vi "Main_FFT.vi"() -> ()   [LabVIEW 2026]
doc: "This template is for the Queued Message Handler design pattern.\n\nThe Event Handling Loop generates messages based on user interface actions.\n\nThe Message Handling Loop processes messages generated by the Event Handling Loop, or by other messages. The messages are string values, so new messages can be added easily to the Message Cases case structure in the Message Handling Loop. Each message cluster can also provide an optional value for Message Data, which is a variant that can be converted to whatever message-specific data is required."
uses:
  SubVIs/Controls/PCO_Config.ctl
  SubVIs/Controls/UI Data.ctl
  SubVIs/pco.labview/camera/Camera.lvclass
  SubVIs/Controls/TypeDef_FGV.ctl
  SubVIs/QMH/Message Queue/Enqueue Message (Single).vi
  SubVIs/QMH/Message Queue/Message Queue.lvlib
  SubVIs/QMH/User Event - Stop/User Event - Stop.lvlib
  SubVIs/pco.labview/pco.sdk/TimingControl/TimingControl.lvlib
panel:
  out "FFT":T1(plugin-control)
  out "Camera":T1(plugin-control)
  in  "# of frames":u16=100
  in  "SavePath":path=path "E:/exp_data/Seb"
  in  "Binning for FFT":u16(ring)=8 items=["1x1"=1, "2x2"=2, "4x4"=4, "8x8"=8]
  in  "Stop live":bool
  in  "FFT?":bool=TRUE
  in  "Grab":bool
  in  "Live":bool
  in  "PCO_Config":T2={"Exposure time (s)"=0.01, "TriggerMode"=0, "ROI X0"=1, "ROI Y0"=1, "ROI X1"=2048, "ROI Y1"=2048, "Binning"=1} {"TriggerMode" items=["auto sequence", "software trigger", "external exposure start", "external exposure control"]}
  out "Current task":string="\"Exit\" button pressed"
  in  "Exit":bool
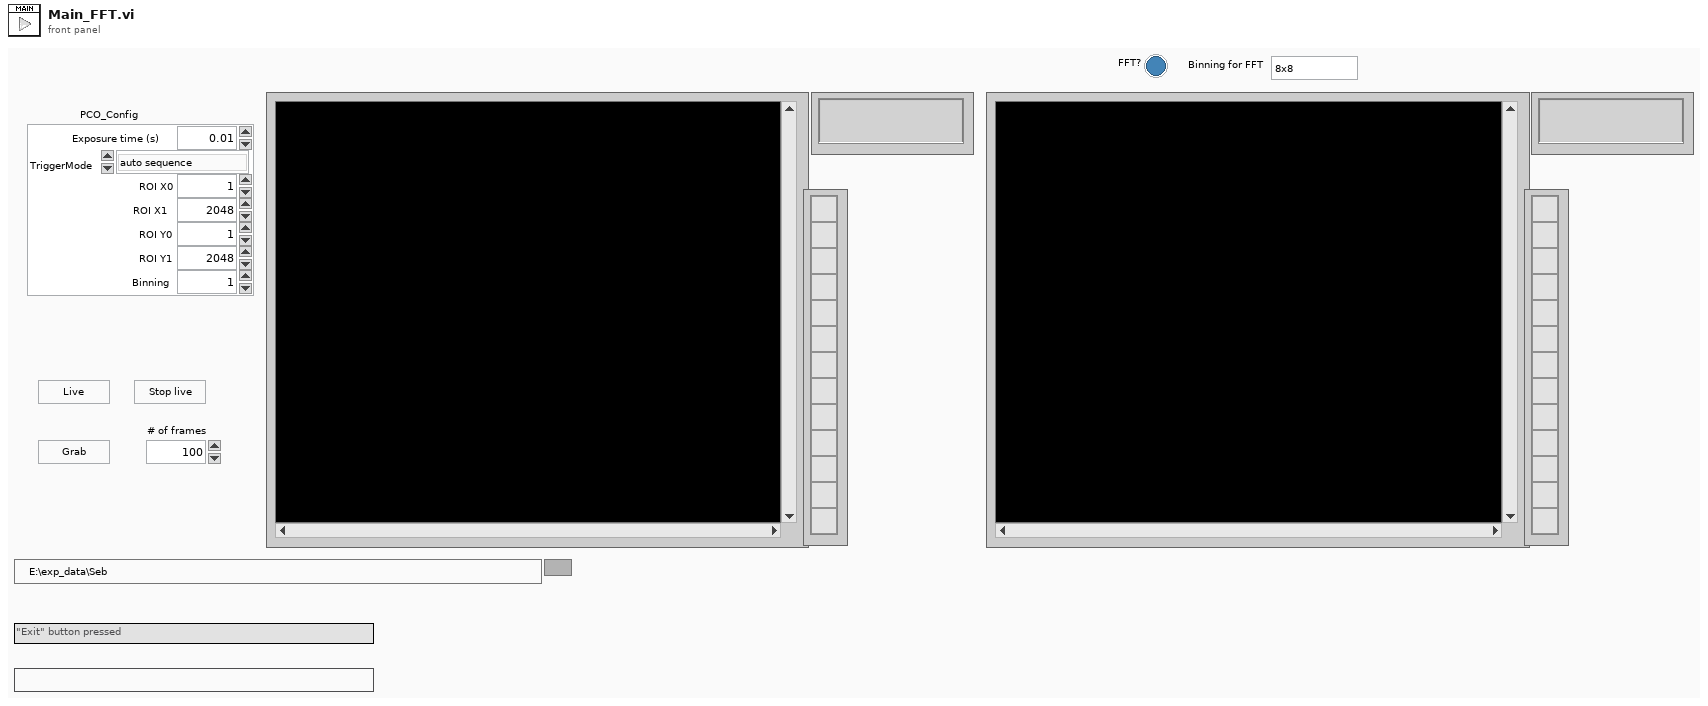
[diagram p1: front panel]
types:
  T1 = typedef "IMAQ Image.ctl" = refnum<image>
  T2 = typedef "PCO_Config.ctl" = cluster{"Exposure time (s)":dbl, "TriggerMode":u16, "ROI X0":u16, "ROI Y0":u16, "ROI X1":u16, "ROI Y1":u16, "Binning":u8}
  T3 = typedef "UI Data.ctl" = cluster{"Data Display Ref":refnum<vi>, "Exit Button Ref":refnum<vi>, "Message":string}
  T4 = typedef "Message Queue.lvlib/All Message Queues.ctl" = cluster{"UI":refnum<queue>, "Camera loop":refnum<queue>, "Display loop":refnum<queue>}
  T5 = typedef "TypeDef_FGV.ctl" = enum16{"Initialize", "Write", "Read"}
  T6 = typedef "Image Type" = u32
  T7 = enum16{"auto sequence", "software trigger", "external exposure start", "external exposure control"}
  T8 = typedef "Camera.lvclass/binning.ctl" = cluster{"vert":u16, "horz":u16, "mode":u16}
  T9 = cluster{"exposure_time_s":dbl, "delay_time_s":dbl, "roi":cluster{"x0":u64, "y0":u64, "x1":u64, "y1":u64}, "timestamp_mode":u16, "pixelrate":u32, "conversion_factor":sgl, "trigger_mode":u16, "acquire_mode":u16, "acquire_sequence_number":u32, "metadata_mode":u16, "noisefilter_mode":u16, "pixel_format":u32, "binning":T8, "auto_exposure":cluster{"region":u16, "min_exposure_s":dbl, "max_exposure_s":dbl}}
  T10 = cluster{"wSignalNum":u16, "wEnabled":u16, "wType":u16, "wPolarity":u16, "wFilterSetting":u16, "wSelected":u16, "dwParameter":u32[], "dwSignalFunctionality":u32[]}
  T11 = cluster{"wVersion":u16, "dwIMAGE_COUNTER":u32, "dwIMAGE_TIME_US":u32, "lvTimestamp":timestamp, "bIMAGE_TIME_STATUS":u8, "wEXPOSURE_TIME_BASE":u16, "dwEXPOSURE_TIME":u32, "dwFRAMERATE_MILLIHZ":u32, "sSENSOR_TEMPERATURE":i16, "wIMAGE_SIZE_X":u16, "wIMAGE_SIZE_Y":u16, "bBINNING_X":u8, "bBINNING_Y":u8, "dwSENSOR_READOUT_FREQUENCY":u32, "wSENSOR_CONV_FACTOR":u16, "dwCAMERA_SERIAL_NO":u32, "wCAMERA_TYPE":u16, "bBIT_RESOLUTION":u8, "bSYNC_STATUS":u8, "wDARK_OFFSET":u16, "bTRIGGER_MODE":u8, "bDOUBLE_IMAGE_MODE":u8, "bCAMERA_SYNC_MODE":u8, "bIMAGE_TYPE":u8, "wCOLOR_PATTERN":u16, "wCAMERA_SUBTYPE":u16, "dwEVENT_NUMBER":u32, "wIMAGE_SIZE_X_Offset":u16, "wIMAGE_SIZE_Y_Offset":u16, "bREADOUT_MODE":u8}[]
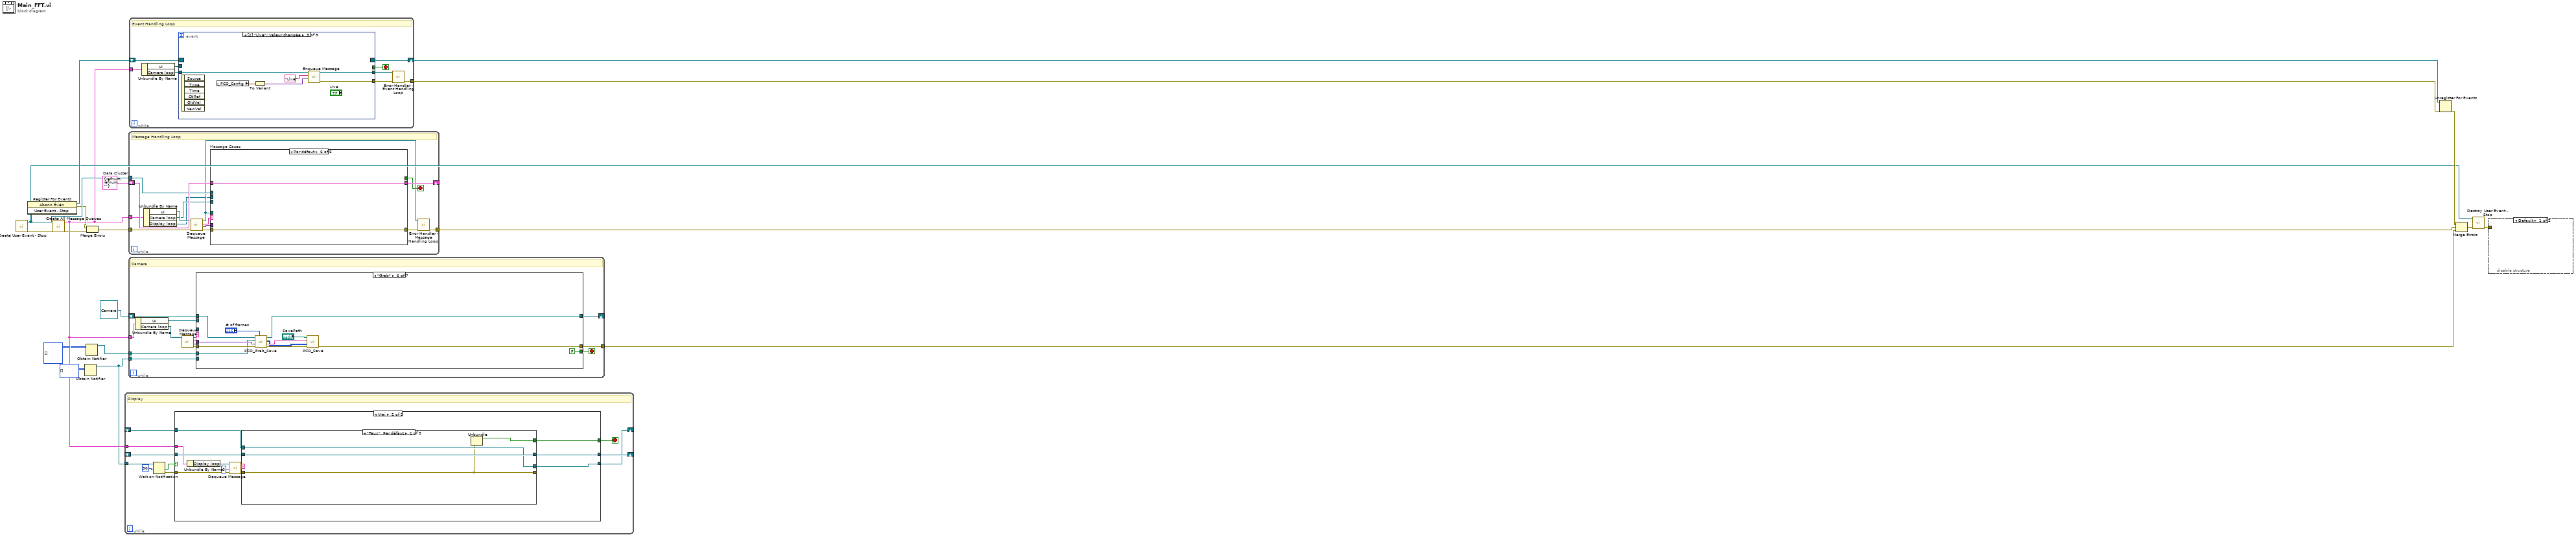
[diagram p0: block diagram]
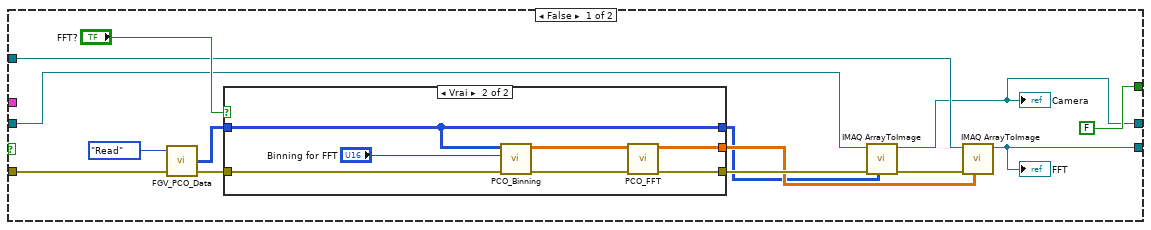
[diagram p2: hidden frame]
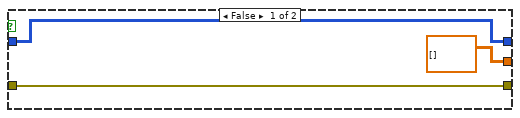
[diagram p3: hidden frame]
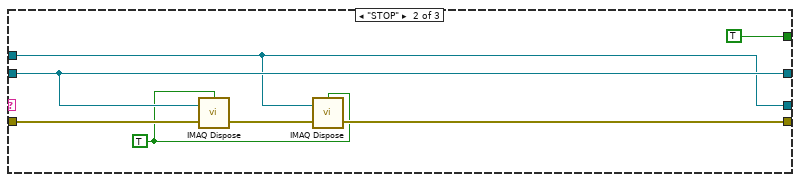
[diagram p4: hidden frame]
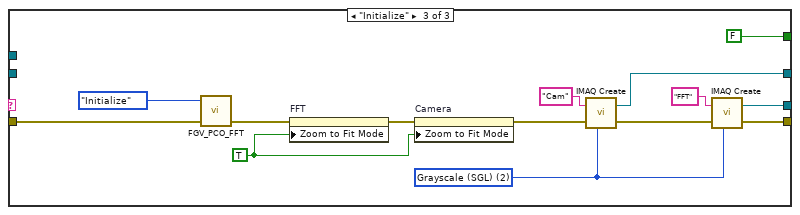
[diagram p5: hidden frame]
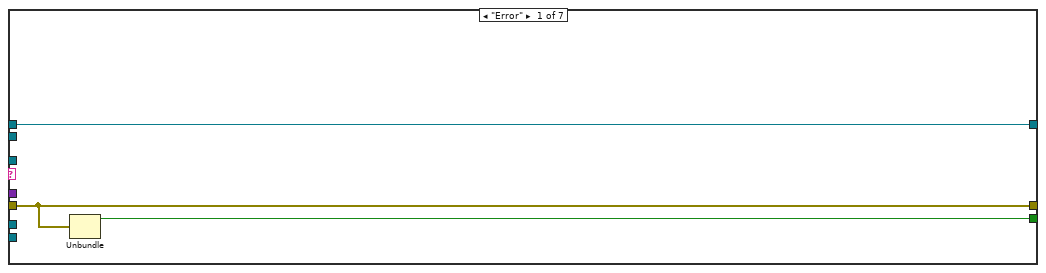
[diagram p6: hidden frame]
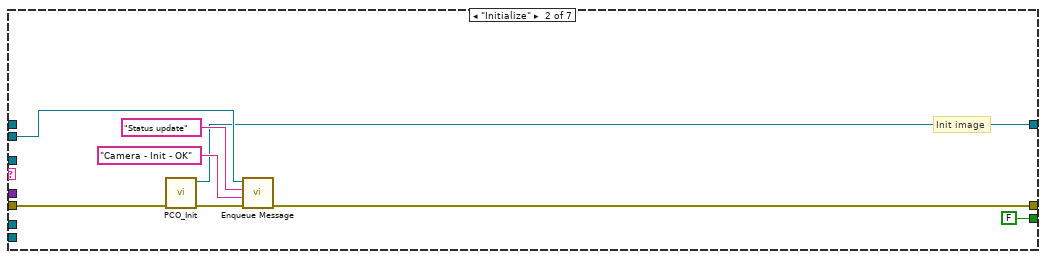
[diagram p7: hidden frame]
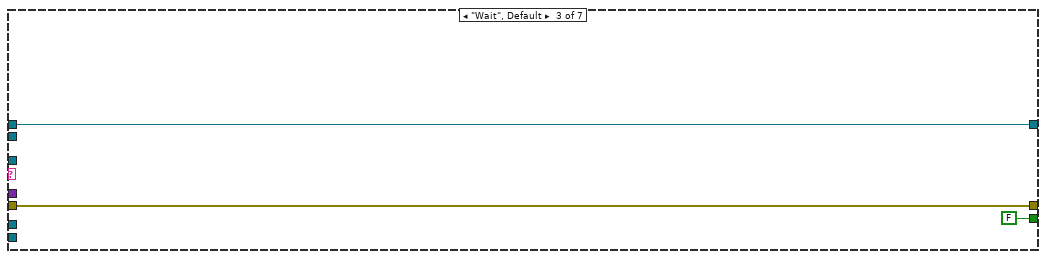
[diagram p8: hidden frame]
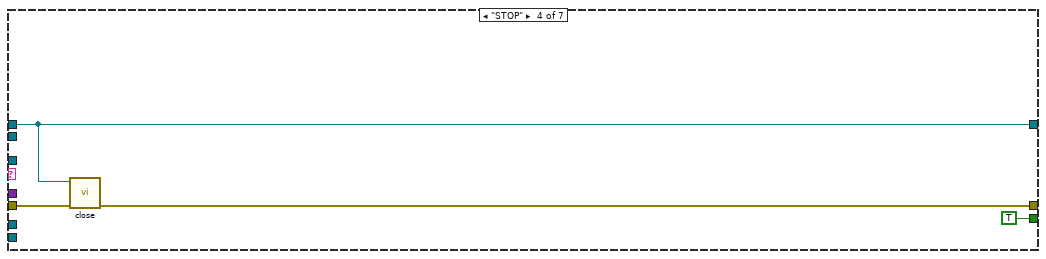
[diagram p9: hidden frame]
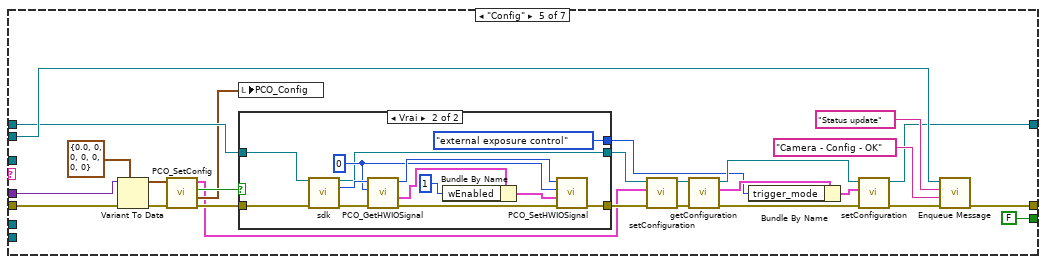
[diagram p10: hidden frame]
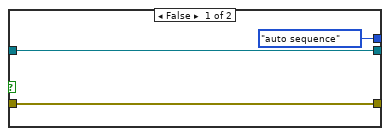
[diagram p11: hidden frame]
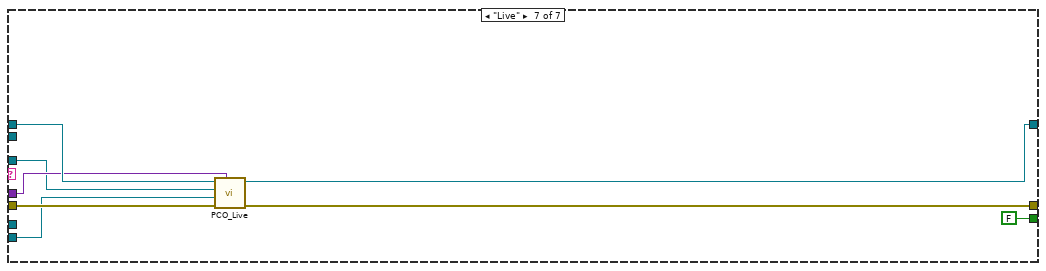
[diagram p12: hidden frame]
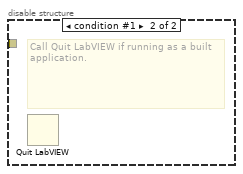
[diagram p13: hidden frame]
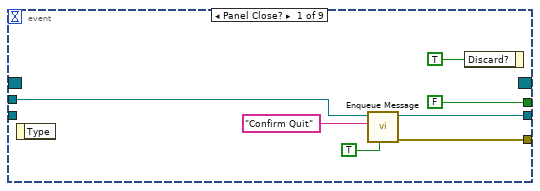
[diagram p14: hidden frame]
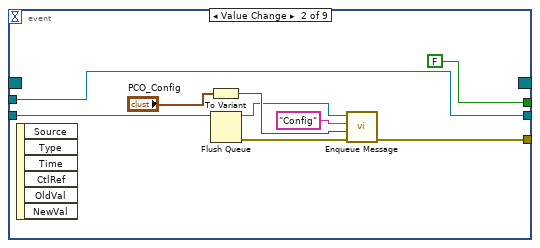
[diagram p15: hidden frame]
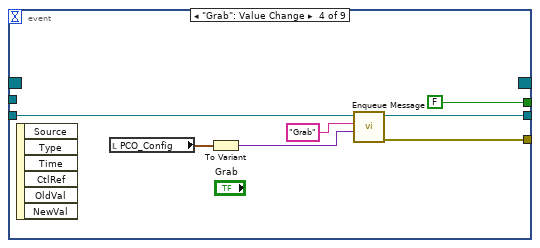
[diagram p16: hidden frame]
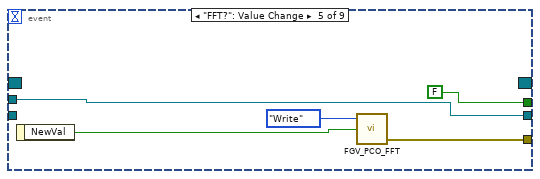
[diagram p17: hidden frame]
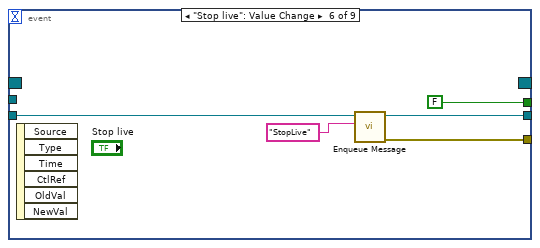
[diagram p18: hidden frame]
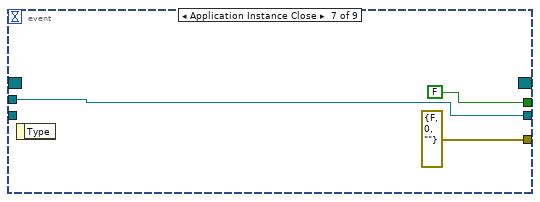
[diagram p19: hidden frame]
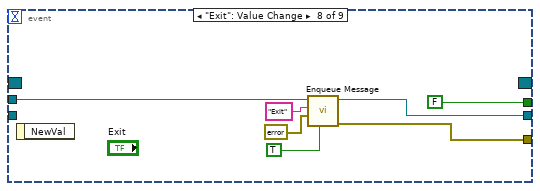
[diagram p20: hidden frame]
diagram:
  w8 = T3 {"Data Display Ref"=refnum, "Exit Button Ref"=refnum, "Message"=""}  # Data Cluster
  n1 = call "Create User Event - Stop.vi"() -> ("error out"=w18:errorcluster, "User Event - Stop"=w11:refnum<user-event>)  [unwired: 10 in]
  n2 = register-events(w11) -> (reference out=w12:refnum<event-registration>, error out=w9:errorcluster)  [unwired: 2 in]
  n3 = call "Create All Message Queues.vi"("error in (no error)"=w18) -> ("error out"=w20:errorcluster, "Message Queues out"=w6:T4)  [unwired: 9 in]
  n4 = Obtain Notifier(notification data type=u16[][] [] ("Graphe d'intensité 2")) -> (notifier out=w1:refnum<notifier>)  [unwired: 3 in, 2 out]
  n5 = Obtain Notifier(notification data type=u16[][][] [] ("Graphe d'intensité 2")) -> (notifier out=w3:refnum<notifier>)  [unwired: 3 in, 2 out]
  n6 = Merge Errors(w9, w20) -> (w10:errorcluster)
  n7 = while {
    tunnel: w6 -> [w30]
    shift-right: [w28] -> _
    shift-left: _ -> [w27]
    shift-right: [w26] -> _
    shift-left: _ -> [w25]
    tunnel: w1 -> [w22]
    stop <- w29 stop-if-true
    # "Display"
    n8 = Wait on Notification(notifier=w22, timeout in ms (-1)=50 ("timeout en ms (-1)")) -> (timed out?=w21:bool, error out=w23:errorcluster)  [unwired: 2 in, 2 out]
    n9 = case shown="Vrai" w21 {
      tunnel: w30 -> [_ w65]
      tunnel: [FALSE w61] -> w29
      tunnel: [w33 w60] -> w28
      tunnel: w27 -> [w32 w59]
      tunnel: [w35 w58] -> w26
      tunnel: w25 -> [w36 w57]
      tunnel: w23 -> [w31 w56]
      frame False {
        n10 = call "FGV_PCO_Data.vi"("error in"=w31, "Action"=TypeDef_FGV."Read") -> ("error out"=w44:errorcluster, "Data"=w43:u16[][])  [unwired: 2 in]
        n11 = case shown="Vrai" "FFT?" {
          tunnel: [w47 w49] -> w41
          tunnel: w44 -> [w47 w54]
          tunnel: w43 -> [w46 w51]
          tunnel: [w46 w51] -> w38
          tunnel: [dbl[][] [] ("FFT") w48] -> w39
          frame False {
          }
          frame True {
            n12 = call "PCO_Binning.vi"("error in"=w54, "Binning"="Binning for FFT", "Data"=w51) -> ("error out"=w53:errorcluster, "Data bin"=w52:dbl[][])  [unwired: 7 in]
            n13 = call "PCO_FFT.vi"("error in (no error)"=w53, "Data"=w52) -> ("error out"=w49:errorcluster, "FFT"=w48:dbl[][])  [unwired: 8 in]
          }
        }
        n14 = call "IMAQ ArrayToImage"("Image Pixels (Float)"=w38, "error in (no error)"=w41, "Image"=w32) -> ("error out"=w40:errorcluster, "Image Out"=w33:T1)  [unwired: 7 in]
        "Camera" <- w33
        n15 = call "IMAQ ArrayToImage"("Image Pixels (Float)"=w39, "error in (no error)"=w40, "Image"=w36) -> ("Image Out"=w35:T1)  [unwired: 7 in, 1 out]
        "FFT" <- w35
      }
      frame True {
        n16 = Unbundle By Name(w65) -> ("Display loop"=w64:refnum<queue>)
        n17 = call "Dequeue Message.vi"("error in (no error)"=w56, "Timeout"=0, "Message Queue"=w64) -> ("error out"=w62:errorcluster, "Message"=w63:string)  [unwired: 5 in, 2 out]
        n18 = case shown="\"Faux\", Par défaut" w63 {
          tunnel: w62 -> [w67 w75 w89]
          tunnel: [w67 w72 w83] -> _
          tunnel: [w66 TRUE FALSE] -> w61
          tunnel: [w69 w74 w86] -> w60
          tunnel: w59 -> [w69 w74 _]
          tunnel: [w68 w71 w84] -> w58
          tunnel: w57 -> [w68 w71 _]
          frame "Faux", Default {
            n19 = Unbundle(w67) -> ("status"=w66:bool)  [unwired: 2 out]
          }
          frame "STOP" {
            w70 = TRUE ("All Images? (No)")
            n20 = call "IMAQ Dispose"("All Images? (No)"=w70, "Image"=w74, "error in (no error)"=w75) -> ("error out"=w73:errorcluster)  [unwired: 3 in]
            n21 = call "IMAQ Dispose"("All Images? (No)"=w70, "Image"=w71, "error in (no error)"=w73) -> ("error out"=w72:errorcluster)  [unwired: 3 in]
          }
          frame "Initialize" {
            w77 = TRUE ("Zoom to Fit Mode")
            w81 = T6 2 items=["Grayscale (U8)", "Grayscale (I16)", "Grayscale (SGL)", "Complex (CSG)", "RGB (U32)", "HSL (U32)", "RGB (U64)", "Grayscale (U16)"] ("Image Type")
            n22 = call "FGV_PCO_FFT.vi"("error in"=w89, "Action"=TypeDef_FGV."Initialize") -> ("error out"=w80:errorcluster)  [unwired: 2 in, 1 out]
            n23 = property on="FFT" class="ImageControl"(error in=w80, "Zoom to Fit Mode"=w77) -> (error out=w79:errorcluster)  [unwired: 1 in, 1 out]
            n24 = property on="Camera" class="ImageControl"(error in=w79, "Zoom to Fit Mode"=w77) -> (error out=w78:errorcluster)  [unwired: 1 in, 1 out]
            n25 = call "IMAQ Create"("Image Name"="Cam", "Image Type"=w81, "error in (no error)"=w78) -> ("New Image"=w86:T1, "error out"=w82:errorcluster)  [unwired: 2 in]
            n26 = call "IMAQ Create"("Image Name"="FFT", "Image Type"=w81, "error in (no error)"=w82) -> ("New Image"=w84:T1, "error out"=w83:errorcluster)  [unwired: 2 in]
          }
        }
      }
    }
  }
  n27 = while {
    tunnel: [w99] -> w7
    tunnel: w6 -> [w98]
    shift-right: [w96] -> _
    shift-left: refnum<class "Camera.lvclass"> refnum ("Camera out") -> [w95]
    tunnel: w3 -> [w92]
    tunnel: w1 -> [w91]
    stop <- w100 stop-if-true
    # "Camera"
    n28 = Unbundle By Name(w98) -> ("UI"=w97:refnum<queue>, "Camera loop"=w93:refnum<queue>)
    n29 = call "Dequeue Message.vi"("Message Queue"=w93) -> ("error out"=w103:errorcluster, "Message Data"=w101:variant, "Message"=w102:string, "dup Message Queue"=w94:refnum<queue>)  [unwired: 7 in]
    n30 = case shown="\"Grab\"" w102 {
      tunnel: w103 -> [w106 w110 w117 w120 w146 w172 w181]
      tunnel: w101 -> [_ _ _ _ w145 w171 w180]
      tunnel: w97 -> [_ w114 _ _ w141 _ _]
      tunnel: [w105 FALSE ("status") FALSE ("status") TRUE FALSE ("status") FALSE ("status") FALSE ("status")] -> w100
      tunnel: [w106 w108 w117 w119 w140 w166 w179] -> w99
      tunnel: w94 -> [_ _ _ _ _ _ w177]
      tunnel: [w104 w109 w116 w118 w128 w175 w178] -> w96
      tunnel: w95 -> [w104 _ w116 w118 w136 w170 w182]
      tunnel: w92 -> [_ _ _ _ _ w164 _]
      tunnel: w91 -> [_ _ _ _ _ _ w176]
      frame "Error" {
        n31 = Unbundle(w106) -> ("status"=w105:bool)  [unwired: 2 out]
      }
      frame "Initialize" {
        # "Init image"
        n32 = call "PCO_Init.vi"("entrée d'erreur (pas d'erreur)"=w110) -> ("sortie d'erreur"=w107:errorcluster, "Camera en sortie"=w109:refnum<class "Camera.lvclass">)  [unwired: 9 in]
        n33 = call-poly "Enqueue Message.vi"("error in (no error)"=w107, "Message Data"="Camera - Init - OK", "Message"="Status update", "Message Queue"=w114) -> ("error out"=w108:errorcluster)  [unwired: 6 in, 1 out]
      }
      frame "Wait", Default {
      }
      frame "STOP" {
        n34 = call-dynamic "close.vi"("error in (no error)"=w120, "Camera in"=w118) -> ("error out"=w119:errorcluster)  [unwired: 9 in]
      }
      frame "Config" {
        n35 = Variant To Data(error in=w146, type=T2 {"Exposure time (s)"=0.0, "TriggerMode"=0, "ROI X0"=0, "ROI Y0"=0, "ROI X1"=0, "ROI Y1"=0, "Binning"=0} ("PCO_Config"), Variant=w145) -> (data=w143:T2, error out=w133:errorcluster)
        n36 = call "PCO_SetConfig.vi"("error in"=w133, "PCO_Config"=w143) -> ("error out"=w132:errorcluster, "PCO_Config 2"=w130:T2, "Trigger externe?"=w134:bool, "configuration"=w122:T9)  [unwired: 6 in]
        n37 = local write "PCO_Config"(w130) -> ()
        n38 = case shown="Vrai" w134 {
          tunnel: w132 -> [w150 w156]
          tunnel: [w150 w151] -> w137
          tunnel: w136 -> [w149 w154]
          tunnel: [w149 w153] -> w135
          tunnel: [T7."auto sequence" ("TriggerMode") T7."external exposure control" ("TriggerMode")] -> w123
          frame False {
          }
          frame True {
            w158 = u16 0 ("wSignalNum")
            n39 = call-dynamic "sdk.vi"("Camera in"=w154, "error in (no error)"=w156) -> ("Camera out"=w153:refnum<class "Camera.lvclass">, "sdk"=w159:u64, "error out"=w155:errorcluster)  [unwired: 11 in]
            n40 = call "PCO_GetHWIOSignal.vi"("error in (no error)"=w155, "wSignalNum"=w158, "ph"=w159) -> ("error out"=w161:errorcluster, "strSignal"=w163:T10, "ph out"=w160:u64)  [unwired: 5 in, 1 out]
            n41 = Bundle By Name(cluster=w163, "wEnabled"=u16 1) -> (w162:T10)
            n42 = call "PCO_SetHWIOSignal.vi"("error in (no error)"=w161, "strSignal"=w162, "wSignalNum"=w158, "ph"=w160) -> ("error out"=w151:errorcluster)  [unwired: 5 in, 2 out]
          }
        }
        n43 = call-dynamic "setConfiguration.vi"("error in (no error)"=w137, "configuration"=w122, "Camera in"=w135) -> ("error out"=w131:errorcluster, "Camera out"=w138:refnum<class "Camera.lvclass">)  [unwired: 7 in]
        n44 = call-dynamic "getConfiguration.vi"("error in (no error)"=w131, "Camera in"=w138) -> ("error out"=w127:errorcluster, "configuration"=w125:T9, "Camera out"=w129:refnum<class "Camera.lvclass">)  [unwired: 7 in]
        n45 = Bundle By Name(cluster=w125, "trigger_mode"=w123) -> (w124:T9)
        n46 = call-dynamic "setConfiguration.vi"("error in (no error)"=w127, "configuration"=w124, "Camera in"=w129) -> ("error out"=w126:errorcluster, "Camera out"=w128:refnum<class "Camera.lvclass">)  [unwired: 7 in]
        n47 = call-poly "Enqueue Message.vi"("error in (no error)"=w126, "Message Data"="Camera - Config - OK", "Message"="Status update", "Message Queue"=w141) -> ("error out"=w140:errorcluster)  [unwired: 6 in, 1 out]
      }
      frame "Grab" {
        n48 = call "PCO_Grab_Save.vi"("# of frames"="# of frames", "entrée d'erreur (pas d'erreur)"=w172, "Message Data"=w171, "notifier out"=w164, "Camera en entrée"=w170) -> ("sortie d'erreur"=w168:errorcluster, "meta_data_list"=w167:T11, "Raw data (U16)"=w165:u16[][][], "Camera en sortie"=w175:refnum<class "Camera.lvclass">)  [unwired: 3 in]
        n49 = call "PCO_Save.vi"("entrée d'erreur (pas d'erreur)"=w168, "raw_image_list (U16)"=w165, "meta_data_list"=w167, "SavePath"="SavePath") -> ("sortie d'erreur"=w166:errorcluster)  [unwired: 7 in]
      }
      frame "Live" {
        n50 = call "PCO_Live.vi"("Message Data"=w180, "entrée d'erreur (pas d'erreur)"=w181, "notifier in"=w176, "dup Message Queue"=w177, "Camera en entrée"=w182) -> ("sortie d'erreur"=w179:errorcluster, "Camera en sortie"=w178:refnum<class "Camera.lvclass">)  [unwired: 5 in]
      }
    }
  }
  n51 = while {
    shift-right: [w197] -> _
    shift-left: w8 -> [w198]
    tunnel: w11 -> [w195]
    tunnel: w10 -> [w194]
    tunnel: [w189] -> w19
    tunnel: w6 -> [w187]
    stop <- w196 stop-if-true
    # "Message Handling Loop"
    n52 = Unbundle By Name(w187) -> ("UI"=w186:refnum<queue>, "Camera loop"=w185:refnum<queue>, "Display loop"=w184:refnum<queue>)
    n53 = call "Dequeue Message.vi"("error in (no error)"=w194, "Message Queue"=w186) -> ("error out"=w193:errorcluster, "Message Data"=w191:variant, "Message"=w192:string, "dup Message Queue"=w190:refnum<queue>)  [unwired: 6 in]
    n54 = case "Message Cases" shown="Par défaut" w192 {
      tunnel: w190 -> [w201 _ _ w223 w237 _]
      tunnel: w193 -> [w206 w212 w219 w225 w238 w246]
      tunnel: [w207 w209 w214 w220 w233 w246] -> w188
      tunnel: w198 -> [w205 w213 w218 w224 w245 w247]
      tunnel: [w204 w213 w218 w224 w245 w247] -> w197
      tunnel: [_ _ _ _ TRUE _] -> w196
      tunnel: w191 -> [_ w211 w217 _ w241 _]
      tunnel: w195 -> [_ _ _ _ w243 _]
      tunnel: w185 -> [_ _ _ _ w236 _]
      tunnel: w184 -> [_ _ _ _ w226 _]
      frame "Initialize" {
        w199 = "Initial Message" ("Initial Message")
        n55 = control-ref of="Current task"() -> (w200:refnum<vi>)
        n56 = control-ref of="Exit"() -> (w203:refnum<vi>)
        n57 = Bundle By Name(cluster=w205, "Data Display Ref"=w200, "Exit Button Ref"=w203, "Message"=w199) -> (w204:T3)
        n58 = call-poly "Enqueue Message.vi"("error in (no error)"=w206, "Message Data"=w199, "Message"="Update Display", "Message Queue"=w201) -> ("error out"=w207:errorcluster)  [unwired: 6 in, 1 out]
      }
      frame "Update Display" {
        n59 = Variant To Data(error in=w212, type="", Variant=w211) -> (data=→"Current task":string, error out=w209:errorcluster)
      }
      frame "Error" {
        n60 = Variant To Data(error in=w219, type=errorcluster {"status"=FALSE, "code"=0, "source"=""} ("error constant"), Variant=w217) -> (data=w215:errorcluster, error out=w214:errorcluster)
        n61 = call <vilib>:"Simple Error Handler.vi"("error in (no error)"=w215) -> ()  [unwired: 4 in, 5 out]
      }
      frame "Confirm Quit" {
        n62 = call-poly "Enqueue Message.vi"("Priority Message? (F)"=TRUE, "error in (no error)"=w225, "Message"="Exit", "Message Queue"=w223) -> ("error out"=w220:errorcluster)  [unwired: 6 in, 1 out]
      }
      frame "Exit" {
        n63 = Variant To Data(error in=w238, type=errorcluster {"status"=FALSE, "code"=0, "source"=""} ("error constant"), Variant=w241) -> (error out=w234:errorcluster)  [unwired: 1 out]
        n64 = Release Queue(queue=w237, error in (no error)=w234) -> (error out=w232:errorcluster)  [unwired: 1 in, 2 out]
        n65 = call-poly "Enqueue Message.vi"("error in (no error)"=w232, "Message"="STOP", "Message Queue"=w236) -> ("error out"=w240:errorcluster, "dup Message Queue"=w239:refnum<queue>)  [unwired: 7 in]
        n66 = Release Queue(queue=w239, error in (no error)=w240) -> (error out=w228:errorcluster)  [unwired: 1 in, 2 out]
        n67 = call-poly "Enqueue Message.vi"("error in (no error)"=w228, "Message"="STOP", "Message Queue"=w226) -> ("error out"=w229:errorcluster, "dup Message Queue"=w230:refnum<queue>)  [unwired: 7 in]
        n68 = Release Queue(queue=w230, error in (no error)=w229) -> (error out=w227:errorcluster)  [unwired: 1 in, 2 out]
        n69 = call "Fire User Event - Stop.vi"("error in (no error)"=w227, "User Event - Stop"=w243) -> ("error out"=w233:errorcluster)  [unwired: 9 in]
      }
      frame Default {
      }
    }
    n70 = call "Error Handler - Message Handling Loop.vi"("error in (no error)"=w188, "Message Queue"=w190) -> ("dup error in"=w189:errorcluster)  [unwired: 8 in, 1 out]
  }
  n71 = while {
    shift-right: [w255] -> w15
    shift-left: w12 -> [w256]
    tunnel: [w251] -> w13
    tunnel: w6 -> [w248]
    stop <- w253 stop-if-true
    # "Event Handling Loop"
    n72 = Unbundle By Name(w248) -> ("UI"=w250:refnum<queue>, "Camera loop"=w249:refnum<queue>)
    n73 = event shown="[2] \"Live\": Valeur changée" {
      selector: w256 -> [_ _ _ _ _ _ _ _ _]
      dyn-events: [_ _ _ _ _ _ _ _ _] -> w255
      timeout: _ -> [_ _ _ _ _ _ _ _ _]
      tunnel: [FALSE ("Discard?") FALSE ("Discard?") _ FALSE ("Discard?") FALSE ("Discard?") FALSE ("Discard?") FALSE ("Discard?") FALSE ("Discard?") TRUE ("Discard?")] -> w253
      tunnel: w250 -> [w262 w272 _ _ w290 _ w298 w305 w309]
      tunnel: [w261 w268 w275 w282 w288 w293 errorcluster {"status"=FALSE, "code"=0, "source"=""} ("error out") w299 errorcluster {"status"=FALSE, "code"=0, "source"=""} ("error out")] -> w254
      tunnel: [w260 w272 w274 w283 w290 w292 w298 w304 w309] -> w252
      tunnel: w249 -> [_ w266 w273 w284 _ w294 _ _ _]
      event Panel Close? {
        n74 = event-data() -> ()  [unwired: 1 in, 1 out]
        n75 = call-poly "Enqueue Message.vi"("Priority Message? (F)"=TRUE, "Message"="Confirm Quit", "Message Queue"=w262) -> ("error out"=w261:errorcluster, "dup Message Queue"=w260:refnum<queue>)  [unwired: 7 in]
        n76 = event-data("Discard?"=TRUE) -> ()  [unwired: 1 in, 1 out]
      }
      event Value Change {
        n77 = event-data() -> ()  [unwired: 1 in, 6 out]
        n78 = To Variant(anything="PCO_Config") -> (Variant=w269:variant)
        n79 = Flush Queue(queue=w266) -> (queue out=w264:refnum<queue>, error out=w265:errorcluster)  [unwired: 1 in, 1 out]
        n80 = call-poly "Enqueue Message.vi"("error in (no error)"=w265, "Message Data"=w269, "Message"="Config", "Message Queue"=w264) -> ("error out"=w268:errorcluster)  [unwired: 6 in, 1 out]
      }
      event "Live": Value Change {
        n81 = event-data() -> ()  [unwired: 1 in, 6 out]
        n82 = local read "PCO_Config"() -> (w278:T2)
        n83 = To Variant(anything=w278) -> (Variant=w277:variant)
        n84 = call-poly "Enqueue Message.vi"("Message Data"=w277, "Message"="Live", "Message Queue"=w273) -> ("error out"=w275:errorcluster, "dup Message Queue"=w274:refnum<queue>)  [unwired: 7 in]
      }
      event "Grab": Value Change {
        n85 = event-data() -> ()  [unwired: 1 in, 6 out]
        n86 = local read "PCO_Config"() -> (w280:T2)
        n87 = To Variant(anything=w280) -> (Variant=w279:variant)
        n88 = call-poly "Enqueue Message.vi"("Message Data"=w279, "Message"="Grab", "Message Queue"=w284) -> ("error out"=w282:errorcluster, "dup Message Queue"=w283:refnum<queue>)  [unwired: 7 in]
      }
      event "FFT?": Value Change {
        n89 = event-data() -> ("NewVal"=w286:bool)  [unwired: 1 in]
        n90 = call "FGV_PCO_FFT.vi"("FFT?"=w286, "Action"=TypeDef_FGV."Write") -> ("error out"=w288:errorcluster)  [unwired: 2 in, 1 out]
      }
      event "Stop live": Value Change {
        n91 = event-data() -> ()  [unwired: 1 in, 6 out]
        n92 = call-poly "Enqueue Message.vi"("Message"="StopLive", "Message Queue"=w294) -> ("error out"=w293:errorcluster, "dup Message Queue"=w292:refnum<queue>)  [unwired: 8 in]
      }
      event Application Instance Close {
        n93 = event-data() -> ()  [unwired: 1 in, 1 out]
      }
      event "Exit": Value Change {
        n94 = event-data() -> ()  [unwired: 1 in, 1 out]
        n95 = call-poly "Enqueue Message.vi"("Priority Message? (F)"=TRUE, "Message Data"=errorcluster {"status"=FALSE, "code"=0, "source"=""} ("error constant"), "Message"="Exit", "Message Queue"=w305) -> ("error out"=w299:errorcluster, "dup Message Queue"=w304:refnum<queue>)  [unwired: 6 in]
      }
      event User Event {
        n96 = event-data() -> ()  [unwired: 1 in, 1 out]
        n97 = local write "Current task"("\"Exit\" button pressed" ("VI Stopped")) -> ()
      }
    }
    n98 = call "Error Handler - Event Handling Loop.vi"("error in (no error)"=w254, "Message Queue"=w252) -> ("dup error in"=w251:errorcluster)  [unwired: 8 in, 1 out]
  }
  n99 = Unregister For Events(event registration refnum=w15, error in=w13) -> (error out=w16:errorcluster)
  n100 = Merge Errors(w16, w19, w7) -> (w17:errorcluster)
  n101 = call "Destroy User Event - Stop.vi"("error in (no error)"=w17, "User Event - Stop"=w11) -> ("error out"=w14:errorcluster)  [unwired: 9 in]
  n102 = disable-structure shown="Default" {
    disable-tunnel: w14 -> [_ _]
    frame condition #0 (active) {
    }
    frame condition #1 {
      # "Call Quit LabVIEW if running as a built application."
      n103 = Quit LabVIEW() -> ()  [unwired: 1 in]
    }
  }
